vi "Wait.vi"(0 "RS232 Port In":refnum<visa-resource-name>="COM1", 1 "Sensor Address In":string="a", 2 "Measurement Type In (Normal)":i32(ring) items=["Normal", "Concurrent", "Continuous"], 3 "Number of Measurements In (1)":i32=1, 4 "Max Acquisition Time (0 sec)":i32, 5 "Error In (No Error)":errorcluster, 6 "CRC (False)":bool, 8 "Parameter In (0)":i32(ring) items=["0", "1", "2", "3", "4", "5", "6", "7", "8", "9"]) -> (10 "Parameter Out":i32(ring) items=["0", "1", "2", "3", "4", "5", "6", "7", "8", "9"], 12 "CRC Out":bool, 14 "RS232 Port Out":refnum<visa-resource-name>="COM1", 15 "Sensor Address Out":string="a", 16 "Measurement Type Out":i32(ring) items=["Normal", "Concurrent", "Continuous"], 17 "Number of Measurements Out":i32, 19 "Error Out":errorcluster)   [LabVIEW 2016, in "SDI-12.lvlib"]
doc: "This VI waits for the sensor to complete the measurement or return a service request. This VI should only be called for Normal and Concurrent Measurements. Do not call with Continuous Measurements."
uses:
  SDI-12.lvlib
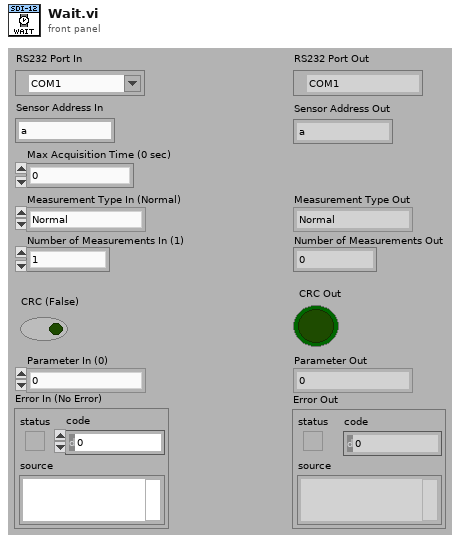
[diagram p1: front panel]
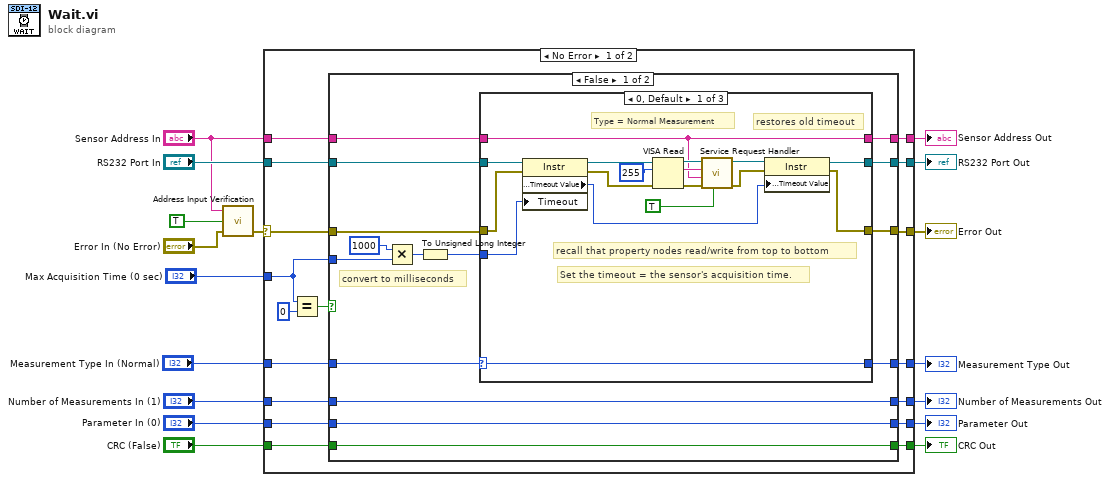
[diagram p0: block diagram]
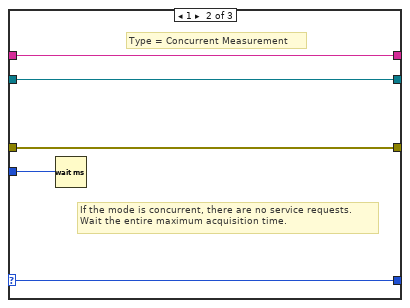
[diagram p2: hidden frame]
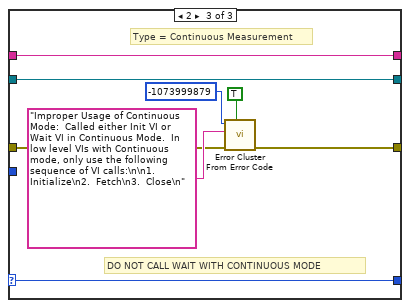
[diagram p3: hidden frame]
diagram:
  n1 = call "Address Input Verification.vi"("Error In (No Error)"="Error In (No Error)", "Error if Bad? (True)"=TRUE ("error if bad? (True)"), "Sensor Address In (a)"="Sensor Address In") -> ("Error Out"=w13:errorcluster)  [unwired: 1 in, 1 out]
  n2 = case shown="No Error" w13 {
    selector: w13 -> [w29 w93]
    tunnel: [w32 w93] -> w17
    tunnel: [w31 w92] -> w16
    tunnel: "RS232 Port In" -> [w30 w92]
    tunnel: "Sensor Address In" -> [w28 w91]
    tunnel: "Number of Measurements In (1)" -> [w27 w90]
    tunnel: [w26 w90] -> w10
    tunnel: "Parameter In (0)" -> [w25 w89]
    tunnel: [w24 w89] -> w8
    tunnel: "CRC (False)" -> [w23 w88]
    tunnel: [w22 w88] -> w6
    tunnel: [w21 w91] -> w5
    tunnel: "Max Acquisition Time (0 sec)" -> [w20 _]
    tunnel: "Measurement Type In (Normal)" -> [w19 w87]
    tunnel: [w18 w87] -> w1
    frame No Error {
      n3 = Equal?(x=w20, y=0) -> (x = y?=w33:bool)
      n4 = case shown="False" w33 {
        tunnel: w20 -> [w44 _]
        tunnel: w29 -> [w49 w86]
        tunnel: [w48 w86] -> w32
        tunnel: w30 -> [w47 w85]
        tunnel: [w46 w85] -> w31
        tunnel: w28 -> [w41 w81]
        tunnel: w27 -> [w40 w84]
        tunnel: [w40 w84] -> w26
        tunnel: w25 -> [w39 w83]
        tunnel: [w39 w83] -> w24
        tunnel: w23 -> [w38 w82]
        tunnel: [w38 w82] -> w22
        tunnel: [w37 w81] -> w21
        tunnel: w19 -> [w36 w80]
        tunnel: [w35 w80] -> w18
        frame False {
          # "convert to milliseconds"
          n5 = Multiply(x=1000, y=w44) -> (x*y=w43:i32)
          n6 = To Unsigned Long Integer(number=w43) -> (unsigned 32bit integer=w42:u32)
          n7 = case shown="0, Default" w36 {
            selector: w36 -> [w50 w67 w72]
            tunnel: w49 -> [w63 w71 w74]
            tunnel: [w54 w71 w75] -> w48
            tunnel: w47 -> [w58 w70 w79]
            tunnel: [w53 w70 w79] -> w46
            tunnel: w42 -> [w52 w69 _]
            tunnel: w41 -> [w51 w68 w73]
            tunnel: [w51 w68 w73] -> w37
            tunnel: [w50 w67 w72] -> w35
            frame 0, Default {
              # "restores old timeout"
              # "recall that property nodes read/write from top to bottom"
              # "Type = Normal Measurement"
              # "Set the timeout = the sensor's acquisition time."
              n8 = property class="Instr"(reference=w58, error in=w63, "Timeout"=w52) -> (reference out=w65:refnum<visa-resource-name>, error out=w64:errorcluster, "General Settings:Timeout Value"=w56:u32)
              n9 = VISA Read(VISA resource name=w65, byte count=u32 255, error in (no error)=w64) -> (VISA resource name out=w62:refnum<visa-resource-name>, read buffer=w61:string, error out=w59:errorcluster)  [unwired: 1 out]
              n10 = call "Service Request Handler.vi"("Check address? (False)"=TRUE ("Check address? (false)"), "Error In (No Error)"=w59, "Expected Sensor Address (a)"=w51, "Service Request"=w61, "RS232 Port In"=w62) -> ("Error Out"=w55:errorcluster, "RS232 Port Out"=w57:refnum<visa-resource-name>)  [unwired: 3 in, 2 out]
              n11 = property class="Instr"(reference=w57, error in=w55, "General Settings:Timeout Value"=w56) -> (reference out=w53:refnum<visa-resource-name>, error out=w54:errorcluster)
            }
            frame 1 {
              # "Type = Concurrent Measurement"
              # "If the mode is concurrent, there are no service requests.  \nWait the entire maximum acquisition time."
              n12 = Wait (ms)(milliseconds to wait=w69) -> ()  [unwired: 1 out]
            }
            frame 2 {
              # "DO NOT CALL WAIT WITH CONTINUOUS MODE"
              # "Type = Continuous Measurement"
              n13 = call <vilib>:"Error Cluster From Error Code.vi"("show call chain? (False)"=TRUE, "error in (no error)"=w74, "error message (\"\")"="Improper Usage of Continuous Mode:  Called either Init VI or Wait VI in Continuous Mode.  In low level VIs with Continuous mode, only use the following sequence of VI calls:\n\n1.  Initialize\n2.  Fetch\n3.  Close\n" ("error message (\"\")"), "error code (0)"=-1073999879 ("error code")) -> ("error out"=w75:errorcluster)  [unwired: 5 in]
            }
          }
        }
        frame True {
          # "If the measurement is already complete, continue to the Fetch phase"
        }
      }
    }
    frame Error {
    }
  }
  "Error Out" <- w17
  "RS232 Port Out" <- w16
  "Parameter Out" <- w8
  "Number of Measurements Out" <- w10
  "CRC Out" <- w6
  "Sensor Address Out" <- w5
  "Measurement Type Out" <- w1
